vi "Pre Launch Init.vi"(11 "Freezer in":refnum<class "Freezer.lvclass">) -> (0 "error out":errorcluster, 3 "Freezer out":refnum<class "Freezer.lvclass">)   [LabVIEW 2015, in "cRIO-Carbondioxide.lvlib" / "CO2-Actor.lvlib" / "Freezer.lvclass"]
doc: "(<B>Filename</B>: Actor Framework.lvlib:Actor.lvclass:Pre Launch Init.vi)\n\nDefines behavior that occurs after the Launch Actor method is invoked but before the actor's Actor Core method begins running.\n\nThe Pre Launch Init method is guaranteed to finish before the Launch Actor method returns to its caller and before the actor itself receives any messages. Any references that the Pre Launch Init method obtains are guaranteed to have the same lifetime as the actor itself. Any errors that the Pre Launch Init method returns will abort the launch.\n\nBy default, this method does nothing. A descendant class may override it to define behavior."
uses:
  Freezer.lvclass
  Freezer.lvclass/Freezer.ctl
  CO2 Actor/CO2 Actor.lvclass
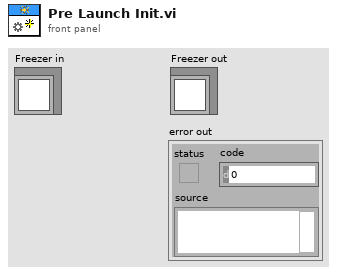
[diagram p1: front panel]
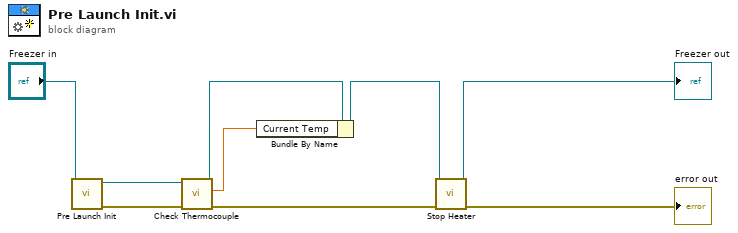
[diagram p0: block diagram]
diagram:
  n1 = call-parent "Pre Launch Init.vi"("CO2 Actor in"="Freezer in") -> ("error out"=w9:errorcluster, "CO2 Actor out"=w7:refnum<class "Freezer.lvclass">)  [unwired: 9 in]
  n2 = call "Check Thermocouple.vi"("error in (no error)"=w9, "Freezer in"=w7) -> ("error out"=w4:errorcluster, "data out"=w6:dbl, "Freezer out"=w5:refnum<class "Freezer.lvclass">)  [unwired: 6 in, 1 out]
  n3 = Bundle By Name(cluster=w5, "Current Temp"=w6) -> (w2:refnum<class "Freezer.lvclass">)
  n4 = call "Stop Heater.vi"("error in (no error)"=w4, "Freezer in"=w2) -> ("error out"=→"error out":errorcluster, "Freezer out"=→"Freezer out":refnum<class "Freezer.lvclass">)  [unwired: 8 in]
